vi "Control Serial.vi"() -> ()   [LabVIEW 2011]
uses:
  <vilib>/Instr/_visa.llb/VISA Configure Serial Port (Instr).vi
panel:
  out "UTC[NIMT]-Cs2":dbl(graph)
  out "UTC[NIMT]-Cs1":dbl(graph)
  out "number 3":dbl format="%#.6e"
  out "number 2":dbl format="%#.6e"
  in  "SR620 Port":refnum<visa-resource-name>
  in  "Control Port":refnum<visa-resource-name>
  out "Humidity":dbl(graph)
  out "Temperature":dbl(graph)
  in  "stop":bool
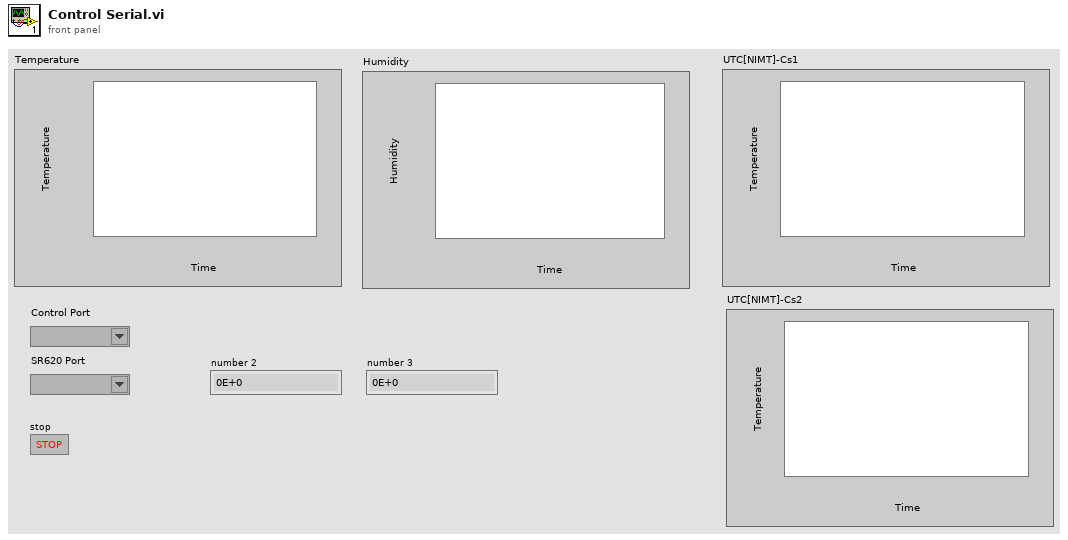
[diagram p1: front panel]
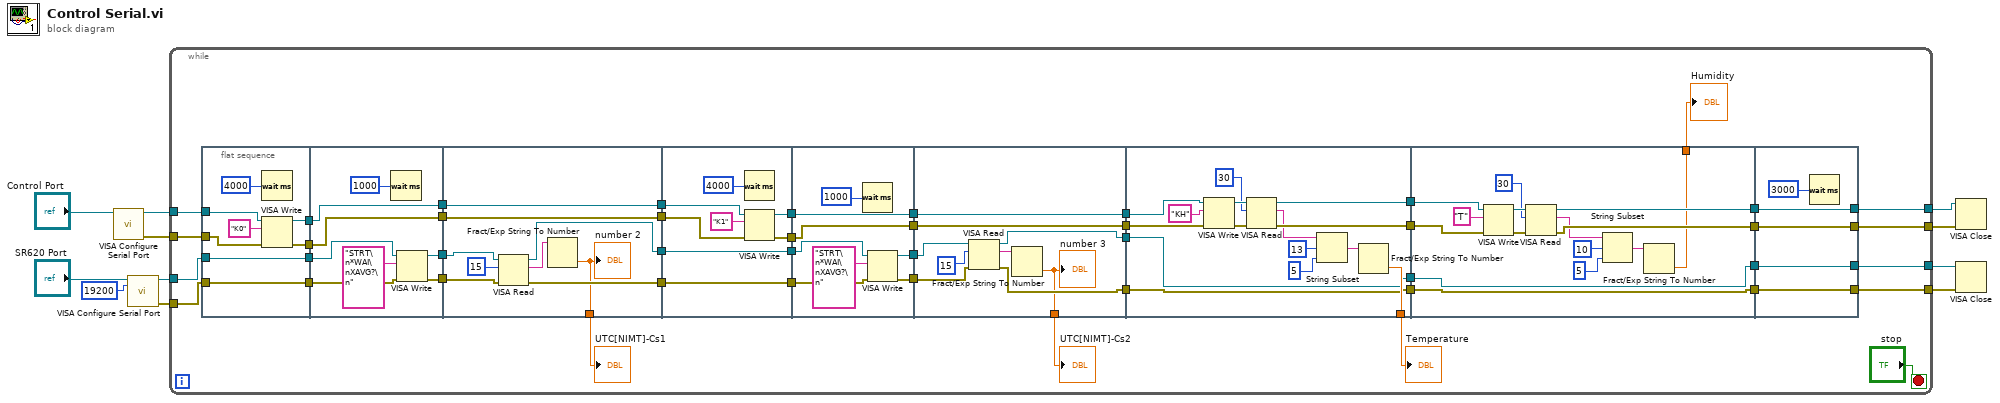
[diagram p0: block diagram]
diagram:
  n1 = call-poly "VISA Configure Serial Port"("VISA resource name"="Control Port") -> ("VISA resource name out"=w11:refnum<visa-resource-name>, "error out"=w10:errorcluster)  [unwired: 13 in]
  n2 = call-poly "VISA Configure Serial Port"("VISA resource name"="SR620 Port", "baud rate (9600)"=u32 19200) -> ("VISA resource name out"=w4:refnum<visa-resource-name>, "error out"=w5:errorcluster)  [unwired: 12 in]
  n3 = while {
    tunnel: w11 -> [w56]
    tunnel: w10 -> [w55]
    tunnel: [w53] -> w9
    tunnel: [w52] -> w8
    tunnel: w5 -> [w43]
    tunnel: w4 -> [w42]
    tunnel: [w38] -> w3
    tunnel: [w36] -> w2
    stop <- "stop" stop-if-true
    n4 = flat-sequence {
      tunnel: w56 -> [w64]
      tunnel: w55 -> [w63]
      tunnel: [w61] -> w33
      tunnel: [w60] -> w31
      tunnel: w43 -> [w58]
      tunnel: w42 -> [w59]
      tunnel: [w59] -> w29
      tunnel: [w58] -> w28
      tunnel: w33 -> [w72]
      tunnel: [w72] -> w32
      tunnel: w31 -> [w71]
      tunnel: [w71] -> w30
      tunnel: w29 -> [w69]
      tunnel: w28 -> [w68]
      tunnel: [w67] -> w27
      tunnel: [w66] -> w26
      tunnel: w32 -> [w81]
      tunnel: [w81] -> w45
      tunnel: w30 -> [w80]
      tunnel: [w80] -> w44
      tunnel: [w78] -> w39
      tunnel: [w77] -> w34
      tunnel: w27 -> [w75]
      tunnel: w26 -> [w74]
      tunnel: [w73] -> w13
      tunnel: w45 -> [w85]
      tunnel: [w83] -> w25
      tunnel: w44 -> [w84]
      tunnel: [w82] -> w24
      tunnel: [w89] -> w23
      tunnel: w39 -> [w89]
      tunnel: [w88] -> w22
      tunnel: w34 -> [w88]
      tunnel: w25 -> [w97]
      tunnel: [w97] -> w21
      tunnel: w24 -> [w96]
      tunnel: [w96] -> w19
      tunnel: w23 -> [w93]
      tunnel: [w92] -> w17
      tunnel: w22 -> [w94]
      tunnel: [w91] -> w16
      tunnel: w21 -> [w106]
      tunnel: [w106] -> w20
      tunnel: w19 -> [w105]
      tunnel: [w105] -> w18
      tunnel: w17 -> [w101]
      tunnel: w16 -> [w102]
      tunnel: [w100] -> w15
      tunnel: [w99] -> w14
      tunnel: [w98] -> w12
      tunnel: w20 -> [w115]
      tunnel: [w113] -> w51
      tunnel: [w112] -> w50
      tunnel: [w111] -> w49
      tunnel: w18 -> [w116]
      tunnel: [w110] -> w40
      tunnel: [w109] -> w35
      tunnel: w15 -> [w109]
      tunnel: w14 -> [w110]
      tunnel: w50 -> [w128]
      tunnel: w49 -> [w127]
      tunnel: [w130] -> w48
      tunnel: [w129] -> w47
      tunnel: [w126] -> w46
      tunnel: [w125] -> w41
      tunnel: w40 -> [w125]
      tunnel: [w124] -> w37
      tunnel: w35 -> [w124]
      tunnel: [w140] -> w52
      tunnel: [w141] -> w53
      tunnel: w48 -> [w141]
      tunnel: w47 -> [w140]
      tunnel: w41 -> [w138]
      tunnel: [w138] -> w38
      tunnel: w37 -> [w137]
      tunnel: [w137] -> w36
      frame #0 {
        n5 = Wait (ms)(milliseconds to wait=u32 4000) -> ()  [unwired: 1 out]
        n6 = VISA Write(VISA resource name=w64, write buffer="K0", error in (no error)=w63) -> (VISA resource name out=w61:refnum<visa-resource-name>, error out=w60:errorcluster)  [unwired: 1 out]
      }
      frame #1 {
        n7 = Wait (ms)(milliseconds to wait=u32 1000) -> ()  [unwired: 1 out]
        n8 = VISA Write(VISA resource name=w69, write buffer="STRT\n*WAI\nXAVG?\n", error in (no error)=w68) -> (VISA resource name out=w66:refnum<visa-resource-name>, error out=w67:errorcluster)  [unwired: 1 out]
      }
      frame #2 {
        n9 = VISA Read(VISA resource name=w74, byte count=u32 15, error in (no error)=w75) -> (VISA resource name out=w77:refnum<visa-resource-name>, read buffer=w76:string, error out=w78:errorcluster)  [unwired: 1 out]
        n10 = Fract/Exp String To Number(string=w76) -> (number=w73:dbl)  [unwired: 3 in, 1 out]
        "number 2" <- w73
      }
      frame #3 {
        n11 = Wait (ms)(milliseconds to wait=u32 4000) -> ()  [unwired: 1 out]
        n12 = VISA Write(VISA resource name=w85, write buffer="K1", error in (no error)=w84) -> (VISA resource name out=w83:refnum<visa-resource-name>, error out=w82:errorcluster)  [unwired: 1 out]
      }
      frame #4 {
        n13 = Wait (ms)(milliseconds to wait=u32 1000) -> ()  [unwired: 1 out]
        n14 = VISA Write(VISA resource name=w94, write buffer="STRT\n*WAI\nXAVG?\n", error in (no error)=w93) -> (VISA resource name out=w91:refnum<visa-resource-name>, error out=w92:errorcluster)  [unwired: 1 out]
      }
      frame #5 {
        n15 = VISA Read(VISA resource name=w102, byte count=u32 15, error in (no error)=w101) -> (VISA resource name out=w100:refnum<visa-resource-name>, read buffer=w103:string, error out=w99:errorcluster)  [unwired: 1 out]
        n16 = Fract/Exp String To Number(string=w103) -> (number=w98:dbl)  [unwired: 3 in, 1 out]
        "number 3" <- w98
      }
      frame #6 {
        n17 = VISA Write(VISA resource name=w115, write buffer="KH", error in (no error)=w116) -> (VISA resource name out=w120:refnum<visa-resource-name>, error out=w121:errorcluster)  [unwired: 1 out]
        n18 = VISA Read(VISA resource name=w120, byte count=u32 30, error in (no error)=w121) -> (VISA resource name out=w112:refnum<visa-resource-name>, read buffer=w107:string, error out=w111:errorcluster)  [unwired: 1 out]
        n19 = String Subset(string=w107, offset (0)=13, length (rest)=5 ("length (rest)")) -> (substring=w108:string)
        n20 = Fract/Exp String To Number(string=w108) -> (number=w113:dbl)  [unwired: 3 in, 1 out]
      }
      frame #7 {
        n21 = VISA Write(VISA resource name=w128, write buffer="T", error in (no error)=w127) -> (VISA resource name out=w134:refnum<visa-resource-name>, error out=w135:errorcluster)  [unwired: 1 out]
        n22 = VISA Read(VISA resource name=w134, byte count=u32 30, error in (no error)=w135) -> (VISA resource name out=w130:refnum<visa-resource-name>, read buffer=w122:string, error out=w129:errorcluster)  [unwired: 1 out]
        n23 = String Subset(string=w122, offset (0)=10, length (rest)=5 ("length (rest)")) -> (substring=w123:string)
        n24 = Fract/Exp String To Number(string=w123) -> (number=w126:dbl)  [unwired: 3 in, 1 out]
      }
      frame #8 {
        n25 = Wait (ms)(milliseconds to wait=u32 3000) -> ()  [unwired: 1 out]
      }
    }
    "Humidity" <- w46
    "Temperature" <- w51
    "UTC[NIMT]-Cs1" <- w13
    "UTC[NIMT]-Cs2" <- w12
  }
  n26 = VISA Close(VISA resource name=w9, error in (no error)=w8) -> ()  [unwired: 1 out]
  n27 = VISA Close(VISA resource name=w2, error in (no error)=w3) -> ()  [unwired: 1 out]
